vi "średnia biegnąca.vi"() -> ()   [LabVIEW 2013]
panel:
  out "Waveform Chart":cluster{"number: 0 to 1":dbl, dbl}(graph)
  out "Ostatnia wartość":dbl
  out "Średnia":dbl
  in  "stop":bool
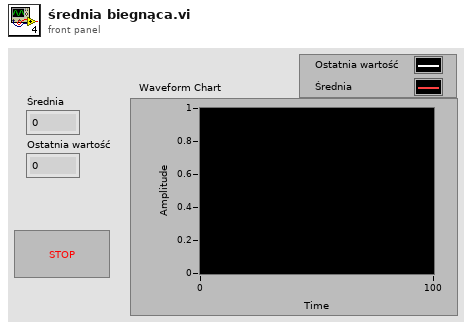
[diagram p1: front panel]
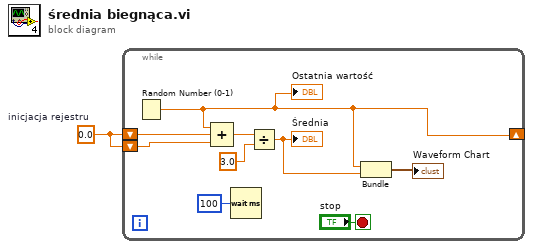
[diagram p0: block diagram]
diagram:
  w1 = 0.0  # inicjacja rejestru
  n1 = while {
    shift-right: [w4] -> _
    shift-left: w1 -> [w9]
    shift-left: w1 -> [w8]
    stop <- "stop" stop-if-true
    n2 = Random Number (0-1)() -> (number: 0 to 1=w4:dbl)
    "Ostatnia wartość" <- w4
    n3 = Compound Arithmetic op=ADD(w4, w9, w8) -> (w7:dbl)
    n4 = Wait (ms)(milliseconds to wait=u32 100) -> ()  [unwired: 1 out]
    n5 = Divide(x=w7, y=3.0) -> (x/y=w3:dbl)
    "Średnia" <- w3
    n6 = Bundle "Bundle"("number: 0 to 1"=w4, w3) -> (→"Waveform Chart":cluster{"number: 0 to 1":dbl, dbl})  [unwired: 1 in]
  }
